vi "AlliGator Save Gate Image Series.vi"(6 "Compress Image in":bool, 8 "error in (no error)":errorcluster, 9 "File Name Format":T1, 10 "Image Array":T2[](array[typedef]), 11 "Folder Path":path) -> (0 "error out":errorcluster, 1 "Message":string)   [LabVIEW 2021, in "AlliGator Files.lvlib"]
doc: "Saves image series (gate images of a FLI Dataset) to a series of TIFF files.\n\nBecause the gate images are floating point data (SGL = floar32), a conversion to 8 or 16 bit images is applied, according to user-set options in the Settings window."
uses:
  AlliGator Files.lvlib
  <vilib>/vision/Image Controls.llb/IMAQ Image.ctl
  AlliGator Settings List.ctl
  AlliGator Exported Image Settings.ctl
  AlliGator Settings.lvlib
  Strings/Strings.lvlib
  Error/Error.lvlib
panel:
  # "see the AlliGator License on the block diagram (Ctrl+E or Window:Show Block Diagram)"
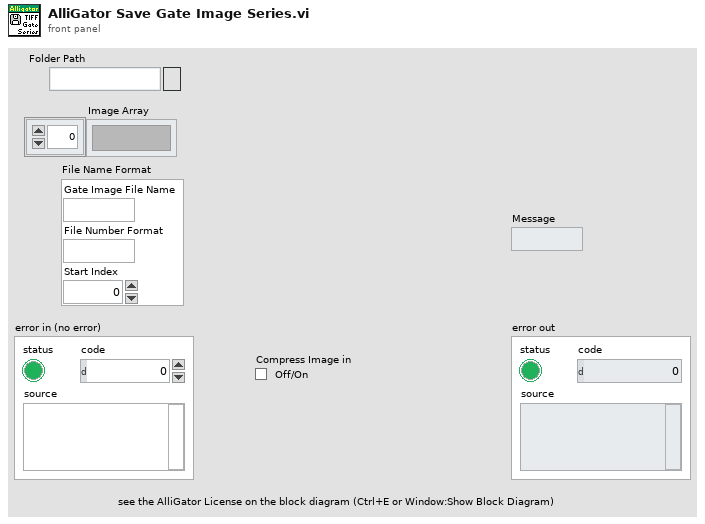
[diagram p1: front panel]
types:
  T1 = cluster{"Gate Image File Name":string, "File Number Format":string, "Start Index":u32}
  T2 = typedef "IMAQ Image.ctl" = refnum<image>
  T3 = typedef "Image Type" = u32
  T4 = typedef "AlliGator Settings.lvlib/AlliGator Exported Image Settings.ctl" = cluster{"bitness":bool, " Min Value":sgl, " Max Value":sgl}
  T5 = typedef "AlliGator Settings.lvlib/AlliGator Settings List.ctl" = enum16{"GUI:Visible Settings Tab", "GUI:Last Run Version", "Source Image:Use Image Histogram for Contrast", "Source Image:Low Count Pixels Rejection Options", "Source Image:High Count Pixels Rejection Options", "Source Image:Use Image Brightness", "Source Image:Blend Overlay with Image Background", "Source Image:Use Fixed ROI Diameter", "Source Image:ROI Diameter", "Source Image:ROI Center Color", "Source Image:Peak Threshold", "Source Image:Intensity Threshold", "Source Image:Image Binning Options", "Source Image:Image Smoothing Options", "Source Image:Image Histogram Active", "Source Image:Invert Binary Mask", "Source Image:Hot Pixel Removal", "Source Image:Overlay Analyzed ROI Center", "Source Image:Auto-Adjust Contrast", "Source Image:Histogram Lower Percentile", "Source Image:Histogram Upper Percentile", "Source Image:Save Source Image", "Source Image:Scale Bar Options", "Source Image:Image Resolution (Pixel Size)", "Source Image:Flatfield Correction", "Source Image:Show Dead Left Columns Correction", "Source Image:Dead Left Columns Correction", "Source Image:Image Pre-Processing Operations Order", "Source Image:Overlay ROI Median", "Source Image:Median Overlay Color", "Data Information:Gate Width", "Data Information:Nanotime Gate Separation", "Data Information:Macrotime Gate Separation", "Data Information:Gate Step", "Data Information:# Gates", "Data Information:Gate Image Exposure", "Data Information:Gate Image Integration", "Data Information:Gates to Skip", "Data Information:Gates to Keep", "Data Information:Define Gates to", "Data Information:Channel Name", "Data Information:Available Channel Names", "Data Information:Channel Arithmetic", "Data Information:Background File Subtraction", "Data Information:Background File", "Data Information:Background Scaling Factor", "Data Information:Background Pile-up Correction", "Data Information:Background Pixel Well Capacity", "Data Information:Laser Period", "Data Information:SYNC Period", "Data Information:Pile-up Correction", "Data Information:Pixel Well Capacity", "Data Information:Dataset Scaling Factor", "Fluorescence Decay_Decay Pre-Processing:Reverse Gates", "Fluorescence Decay_Decay Pre-Processing:Verbose Decay Pre-Processing", "Fluorescence Decay_Decay Pre-Processing:Use Decay Pre-Processing", "Fluorescence Decay_Decay Pre-Processing:Background Subtraction", "Fluorescence Decay_Decay Pre-Processing:Background Definition Range", "Fluorescence Decay_Decay Pre-Processing:Baseline Subtraction Method", "Fluorescence Decay_Decay Pre-Processing:Decay Pre-Processing Operations Order", "Fluorescence Decay_Decay Pre-Processing:Smoothing Parameter", "Fluorescence Decay_Decay Pre-Processing:Shift Decay", "Fluorescence Decay_Decay Pre-Processing:Decay Shift Parameters", "Fluorescence Decay_Decay Pre-Processing:Fold Decay", "Fluorescence Decay_Decay Pre-Processing:# Folds", "Fluorescence Decay_Decay Pre-Processing:1-Normalize Decay", "Fluorescence Decay_Decay Pre-Processing:[0-1]-Normalize Decay", "Fluorescence Decay_Decay Pre-Processing:Smoothen Decay", "Fluorescence Decay_Decay Pre-Processing:Extrapolate Decay", "Fluorescence Decay_Decay Pre-Processing:Use Periodicity", "Fluorescence Decay_Decay Pre-Processing:Use Cursors", "Fluorescence Decay_Decay Pre-Processing:Tail Fraction", "Fluorescence Decay_Decay Pre-Processing:Head Fraction", "Fluorescence Decay_Decay Pre-Processing:Additional Points", "Fluorescence Decay_Decay Pre-Processing:Straighten Decay", "Fluorescence Decay_Decay Pre-Processing:Constant Background", "Fluorescence Decay_Decay Pre-Processing:Pixel-Normalize Decay", "Fluorescence Decay_Advanced Analysis:Extract IRF instead of Decay", "Fluorescence Decay_Advanced Analysis:IRF Extraction Options", "Fluorescence Decay_Advanced Analysis:IRF Optimization Options", "Fluorescence Decay_Advanced Analysis:Square Pulse Options", "Fluorescence Decay_Advanced Analysis:IRF Order", "Fluorescence Decay_Advanced Analysis:IRF Time Constants", "Fluorescence Decay_Advanced Analysis:Wavelet Analysis Options", "Fluorescence Decay_Advanced Analysis:Average Lifetime Options", "Fluorescence Decay_Fit Options:Fit Options", "Fluorescence Decay_Fit Options:Use Legacy Fitting Approach", "Fluorescence Decay_Fit Options:Use Data Information Laser Period", "Fluorescence Decay_Fit Parameters:Displayed Fit Parameters", "Fluorescence Decay_Fit Parameters:Fit Parameter Constraints", "Fluorescence Decay_Fit Parameters:Export Tabulated Results", "Fluorescence Decay_Fit Parameters:MLE Baseline Offset Type", "Fluorescence Decay_Fit Parameters:MLE Baseline Offset", "Fluorescence Decay_Fit Parameters:Guess Parameter Names", "Fluorescence Decay_Fit Parameters:Guess Parameter Values", "Fluorescence Decay_Fit Parameters:Guess Parameters Options", "Fluorescence Decay_Styles:Show Last Decay Only", "Fluorescence Decay_Styles:Decay Graph Color Array", "Fluorescence Decay:Decay Graph Active", "Fluorescence Decay Statistics:Min Peak Value", "Fluorescence Decay Statistics:Reject Low Decay Peak Pixels", "Fluorescence Decay Statistics:Reject High Decay Peak Pixels", "Fluorescence Decay Statistics:Max Peak Value", "Time Traces:Use File Timestamp", "Time Traces:Time Step", "Time Traces:Use Intensity Correction File", "Time Traces:Intensity Correction File", "Phasor Plot:Phasor Plot Smoothing Options", "Phasor Plot:Phasor Plot Size", "Phasor Plot:Phasor Plot Graphics Options", "Phasor Plot:Cumulative Phasor Plot", "Phasor Plot:Use Phasor Brightness", "Phasor Plot:Blend Overlay with Phasor Background", "Phasor Plot:Save Phasor Plot", "Phasor Plot:Show References", "Phasor Plot:Phasor Ratio Decay Range", "Phasor Plot:Exponential Fading", "Phasor Plot:Phasor Ratio Reference Colors", "Phasor Plot:Reference Radius", "Phasor Plot:Show Color Map Vertices", "Phasor Plot:Phasor Plot Active", "Phasor Plot:Phasor Ratio Color Map Type", "Phasor Plot:Phasor Ratio Color Map", "Phasor Plot:Phasor Ratio Display Range", "Phasor Plot:Selected Image ROI(s)", "Phasor Plot:All Image ROIs", "Phasor Plot:Selected Phasor Plot ROI(s)", "Phasor Plot:All Phasor Plot ROIs", "Phasor Plot:Phasor Ratio Color-Coded Quantity", "Phasor Plot:Store Phasor Harmonics", "Phasor Plot:Draw Reference Segment", "Phasor Plot:User-Defined Quantity", "Phasor Graph:Phasor Frequency", "Phasor Graph:Phasor Ratio Type", "Phasor Graph:Pixel-level Phasor Computation", "Phasor Graph:Save Phasor Graph", "Phasor Graph:Phasor Graph Active", "Phasor Graph:Phasor SDV Options", "Phasor Calibration:Use Backup Calibration if needed", "Phasor Graph:Define Shortest Lifetime as", "Phasor Calibration:Backup Calibration Type", "Phasor Calibration:Calibration Type", "Phasor Calibration:Calibration Lifetime", "Phasor Calibration:Calibration Map Algorithm", "Single-Exponential Phasor Locus (SEPL):Gate Parameters", "Single-Exponential Phasor Locus (SEPL):User-defined Gate", "Single-Exponential Phasor Locus (SEPL):User-defined IRF", "Single-Exponential Phasor Locus (SEPL):Phasor Parameters", "Single-Exponential Phasor Locus (SEPL):Decay & IRF Parameters", "Single-Exponential Phasor Locus (SEPL):Display Parameters", "Lifetime Analysis:Decay Analysis Parameters", "Lifetime Analysis:Lifetime Map Active", "Plugins:Python Settings", "Miscellaneous:Verbose Mode", "Miscellaneous:Beep after Script", "Miscellaneous:Saved Image File Format", "Miscellaneous:Exported Gate Image Settings", "Miscellaneous:Include Loading in Timing", "Miscellaneous:Verbose Settings Mode", "Miscellaneous:Histogram Options", "Miscellaneous:Beep on Error", "Miscellaneous:# Logical Processors Used", "Miscellaneous:ROI Description Max Characters", "Miscellaneous:Verbose Error Mode", "Miscellaneous:Transparent Mask Color"}
  T6 = cluster{"Rows Per Strip":i32, "Photometric":i32, "Compression Type":i32}
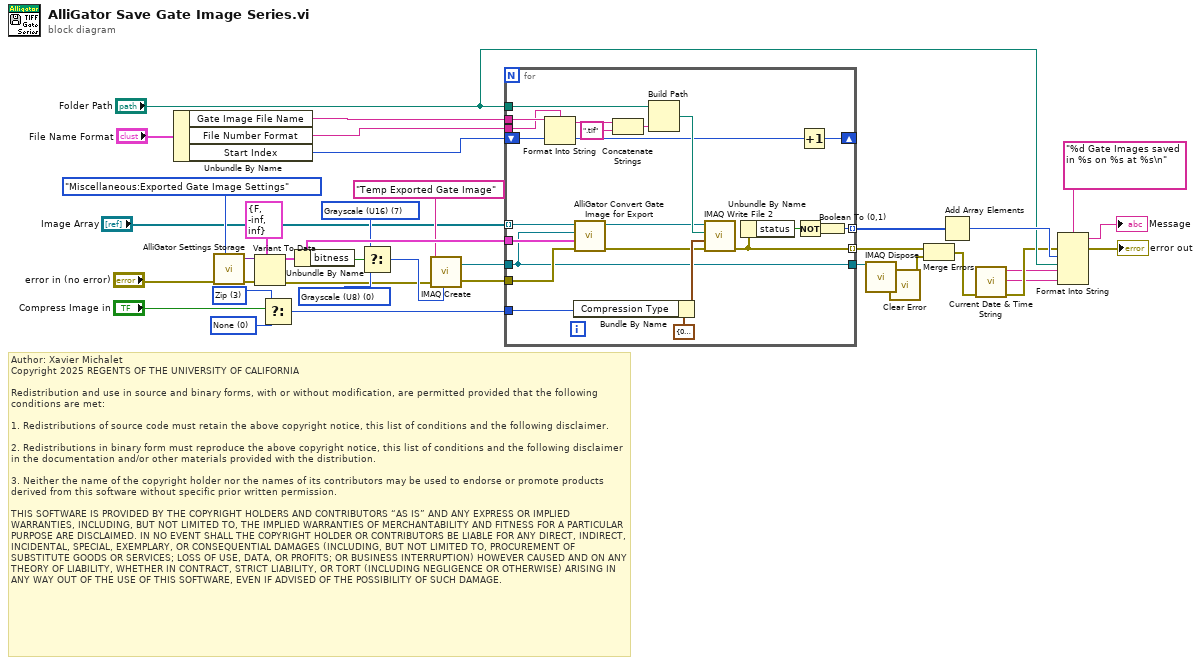
[diagram p0: block diagram]
diagram:
  w31 = T3 7 items=["Grayscale (U8)", "Grayscale (I16)", "Grayscale (SGL)", "Complex (CSG)", "RGB (U32)", "HSL (U32)", "RGB (U64)", "Grayscale (U16)"] ("Image Type")
  w30 = T3 0 items=["Grayscale (U8)", "Grayscale (I16)", "Grayscale (SGL)", "Complex (CSG)", "RGB (U32)", "HSL (U32)", "RGB (U64)", "Grayscale (U16)"] ("Image Type")
  w15 = 0 items=["None", "JPEG", "Run Length Encoded", "Zip"] ("Compression Type")
  w16 = 3 items=["None", "JPEG", "Run Length Encoded", "Zip"] ("Compression Type")
  # "Author: Xavier Michalet\nCopyright 2025 REGENTS OF THE UNIVERSITY OF CALIFORNIA\n\nRedistribution and use in source and binary forms, with or without modification, are permitted provided that the following conditions are met:\n\n1. Redistributions of source code must retain the above copyright notice, this list of conditions and the following disclaimer.\n\n2. Redistributions in binary form must reproduce the above copyright notice, this list of conditions and the following disclaimer in the documentation and/or other materials provided with the distribution.\n\n3. Neither the name of the copyright holder nor the names of its contributors may be used to endorse or promote products derived from this software without specific prior written permission.\n\nTHIS SOFTWARE IS PROVIDED BY THE COPYRIGHT HOLDERS AND CONTRIBUTORS “AS IS” AND ANY EXPRESS OR IMPLIED WARRANTIES, INCLUDING, BUT NOT LIMITED TO, THE IMPLIED WARRANTIES OF MERCHANTABILITY AND FITNESS FOR A PARTICULAR PURPOSE ARE DISCLAIMED. IN NO EVENT SHALL THE COPYRIGHT HOLDER OR CONTRIBUTORS BE LIABLE FOR ANY DIRECT, INDIRECT, INCIDENTAL, SPECIAL, EXEMPLARY, OR CONSEQUENTIAL DAMAGES (INCLUDING, BUT NOT LIMITED TO, PROCUREMENT OF SUBSTITUTE GOODS OR SERVICES; LOSS OF USE, DATA, OR PROFITS; OR BUSINESS INTERRUPTION) HOWEVER CAUSED AND ON ANY THEORY OF LIABILITY, WHETHER IN CONTRACT, STRICT LIABILITY, OR TORT (INCLUDING NEGLIGENCE OR OTHERWISE) ARISING IN ANY WAY OUT OF THE USE OF THIS SOFTWARE, EVEN IF ADVISED OF THE POSSIBILITY OF SUCH DAMAGE."
  n1 = Unbundle By Name("File Name Format") -> ("Gate Image File Name"=w10:string, "File Number Format"=w8:string, "Start Index"=w9:u32)
  n2 = call "AlliGator Settings Storage.vi"("AlliGator Settings List"=AlliGator_Settings_List."Miscellaneous:Exported Gate Image Settings", "Error In"="error in (no error)") -> ("Error Out"=w24:errorcluster, "Variant Data out"=w25:variant)  [unwired: 8 in]
  n3 = Variant To Data(error in=w24, type=T4 {"bitness"=FALSE, " Min Value"=-inf, " Max Value"=inf} ("Exported Gate Image Settings"), Variant=w25) -> (data=w35:T4, error out=w28:errorcluster)
  n4 = Select(t=w16, s="Compress Image in", f=w15) -> (s? t:f=w17:i32)
  n5 = Unbundle By Name(w35) -> ("bitness"=w27:bool)
  n6 = Select(t=w31, s=w27, f=w30) -> (s? t:f=w32:T3)
  n7 = call "IMAQ Create"("Image Name"="Temp Exported Gate Image", "Image Type"=w32, "error in (no error)"=w28) -> ("New Image"=w33:T2, "error out"=w34:errorcluster)  [unwired: 2 in]
  n8 = for {
    tunnel: "Image Array" -> [w43] mode=indexing
    tunnel: [w54] -> w13 mode=indexing
    tunnel: w17 -> [w57]
    tunnel: "Folder Path" -> [w56]
    tunnel: [w52] -> w21 mode=indexing
    tunnel: w10 -> [w50]
    shift-right: [w46] -> _
    shift-left: w9 -> [w47]
    tunnel: w8 -> [w49]
    tunnel: w33 -> [w40]
    tunnel: w34 -> [w44]
    tunnel: w35 -> [w41]
    tunnel: [w40] -> w36
    n9 = Format Into String(format string=w49, initial string=w50, w47) -> (resulting string=w48:string)  [unwired: 1 in, 1 out]
    n10 = Bundle By Name(cluster=T6 {"Rows Per Strip"=0, "Photometric"=1, "Compression Type"=0} ("TIFF Options"), "Compression Type"=w57) -> (w58:T6)
    n11 = call "AlliGator Convert Gate Image for Export.vi"("error in (no error)"=w44, "Exported Gate Image Settings"=w41, "Dest Image"=w40, "Original Image"=w43) -> ("error out"=w45:errorcluster, "Result Image"=w42:T2)  [unwired: 6 in]
    n12 = Concatenate Strings(w48, ".tif" ("string")) -> (w39:string)
    n13 = Build Path(base path=w56, name or relative path=w39) -> (appended path=w55:path)
    n14 = call-poly "IMAQ Write File 2"("error in (no error)"=w45, "TIFF Options"=w58, "File Path"=w55, "Image"=w42) -> ("error out"=w54:errorcluster)  [unwired: 6 in, 1 out]
    n15 = Unbundle By Name(w54) -> ("status"=w53:bool)
    n16 = Not(x=w53) -> (.not. x?=w51:bool)
    n17 = Increment(x=w47) -> (x+1=w46:u32)
    n18 = Boolean To (0,1)(Boolean=w51) -> (0, 1=w52:i16)
  }
  n19 = call "IMAQ Dispose"("Image"=w36) -> ("error out"=w2:errorcluster)  [unwired: 5 in]
  n20 = call "Clear Error.vi"("Error In"=w2) -> ("no Error Out"=w1:errorcluster)  [unwired: 8 in]
  n21 = Merge Errors(w13, w1) -> (w6:errorcluster)
  n22 = Add Array Elements(numeric array=w21) -> (sum=w22:i16)
  n23 = call "Current Date & Time String.vi"("Error In"=w6) -> ("Error Out"=w5:errorcluster, "time string"=w3:string, "date string"=w4:string)  [unwired: 8 in]
  n24 = Format Into String(format string="%d Gate Images saved in %s on %s at %s\n", error in=w5, w22, "Folder Path", w4, w3) -> (resulting string=→"Message":string, error out=→"error out":errorcluster)  [unwired: 1 in]
